vi "Implemeted_Discrete_Controller.vi"(6 "Loop Itr":i32, 8 "Other variables":T1, 9 "systems":T6 {"SysD"."Transport Delay" format="%.2f"; "SysD"."D" format="%#.2g"; "SysD"."C" format="%#.2g"; "SysD"."B" format="%#.2g"; "SysD"."A" format="%#.2g"; "SysD"."properties"."Sampling Time" format="%#.6p"; "SysD"."properties"."Output Delays" format="%.4f"; "SysD"."properties"."Input Delays" format="%.4f"; "sysDo"."Transport Delay" format="%.2f"; "sysDo"."D" format="%#.2g"; "sysDo"."C" format="%#.2g"; "sysDo"."B" format="%#.2g"; "sysDo"."A" format="%#.2g"; "sysDo"."properties"."Sampling Time" format="%#.6p"; "sysDo"."properties"."Output Delays" format="%.4f"; "sysDo"."properties"."Input Delays" format="%.4f"; "sysDi"."Transport Delay" format="%.2f"; "sysDi"."D" format="%#.2g"; "sysDi"."C" format="%#.2g"; "sysDi"."B" format="%#.2g"; "sysDi"."A" format="%#.2g"; "sysDi"."properties"."Sampling Time" format="%#.6p"; "sysDi"."properties"."Output Delays" format="%.4f"; "sysDi"."properties"."Input Delays" format="%.4f"; "sysDC"."transfer function(s)"."delay" format="%.4f"; "sysDC"."transfer function(s)"."Denominator" format="%#_3g"; "sysDC"."transfer function(s)"."Numerator" format="%#_3g"; "sysDC"."properties"."Sampling Time" format="%#.6p"; "sysDC"."properties"."Output Delays" format="%.4f"; "sysDC"."properties"."Input Delays" format="%.4f"}, 10 "Lean Angle":dbl, 11 "Steer Angle":dbl format="%#_13g") -> (2 "Direction":dbl, 3 "Duty Cycle":dbl, 4 "Loop Out":i32)   [LabVIEW 2016]
uses:
  <vilib>/addons/Control Design/_Model Construction/Model Typedefs.llb/CD State Space Model (MIMO).ctl
  <vilib>/addons/Control Design/_Model Construction/Model Typedefs.llb/CD General Elements.ctl
  <vilib>/addons/Control Design/_Model Construction/Model Typedefs.llb/CD Transfer Function Model (MIMO).ctl
  <vilib>/addons/Control Design/_Model Construction/Model Typedefs.llb/CD Transfer Function Model (SISO).ctl
  <vilib>/Analysis/Matrix/Datatypes/RealMatrix.ctl
  <vilib>/Simulation/DiscreteLinear/Implementation/NILVSim Discrete Transfer Function Direct.llb/SIM Discrete Transfer Function Diagram (SISO).vi
  <vilib>/Analysis/baseanly.llb/Real A x B.vi
  <vilib>/Simulation/ContinuousLinear/Implementation/Shared/SIM Transfer Function Support.llb/SIM TransferFunction Normalize to Buffer.vi
  <vilib>/Simulation/DiscreteLinear/Implementation/Shared/SIM Init Discrete States.vi
  <vilib>/Simulation/DiscreteLinear/Implementation/NILVSim Discrete Transfer Function Direct.llb/SIM Transfer Function Direct core (SISO).vi
  <vilib>/Simulation/ContinuousLinear/Implementation/Shared/SIM Transfer Function Support.llb/SIM TransferFunction Normalize.vi
  <vilib>/Simulation/Implementation/Shared/SIM Polynomials.llb/SIM Remove Zero Coefficients (DBL).vi
  <vilib>/Simulation/Implementation/Shared/SIM Polynomials.llb/SIM Divide Polynomials (DBL).vi
  <vilib>/Simulation/Implementation/Shared/SIM BuildSimErr.vi
  <vilib>/Analysis/Matrix/Numeric/Conversions/Matrix To Array - RM.vi
  <vilib>/imath/engines/lvmath2/RunTimeEngine/NodeEndStatement/NIMS_NodeEndStatement_Output.vi
  <instcachedir>/0/NIMS_NodeEndStatement_Output_53EC0D466D134D7ABD903AC30B43404B.lvgen/NIMS_NodeEndStatement_Output_53EC0D466D134D7ABD903AC30B43404B_002.vi
  <vilib>/imath/engines/lvmath2/RunTimeEngine/ErrorHandling/NIMS_Finalize Error.vi
  <vilib>/Analysis/Matrix/Numeric/Subtract/Subtract (Elementwise) - R,RM.vi
  <vilib>/Analysis/Matrix/Numeric/Add/Add - RM,RM.vi
  <vilib>/Simulation/Implementation/XNodeFramework/SimXNode/SimX.xnode
  <vilib>/Analysis/NI_AALBase.lvlib
  <vilib>/Analysis/Matrix/NI_Matrix.lvlib
  <vilib>/addons/Control Design/_Model Construction/NI_LinSys_Model Typedefs.lvlib
panel:
  # "Inputs"
  # "Outputs"
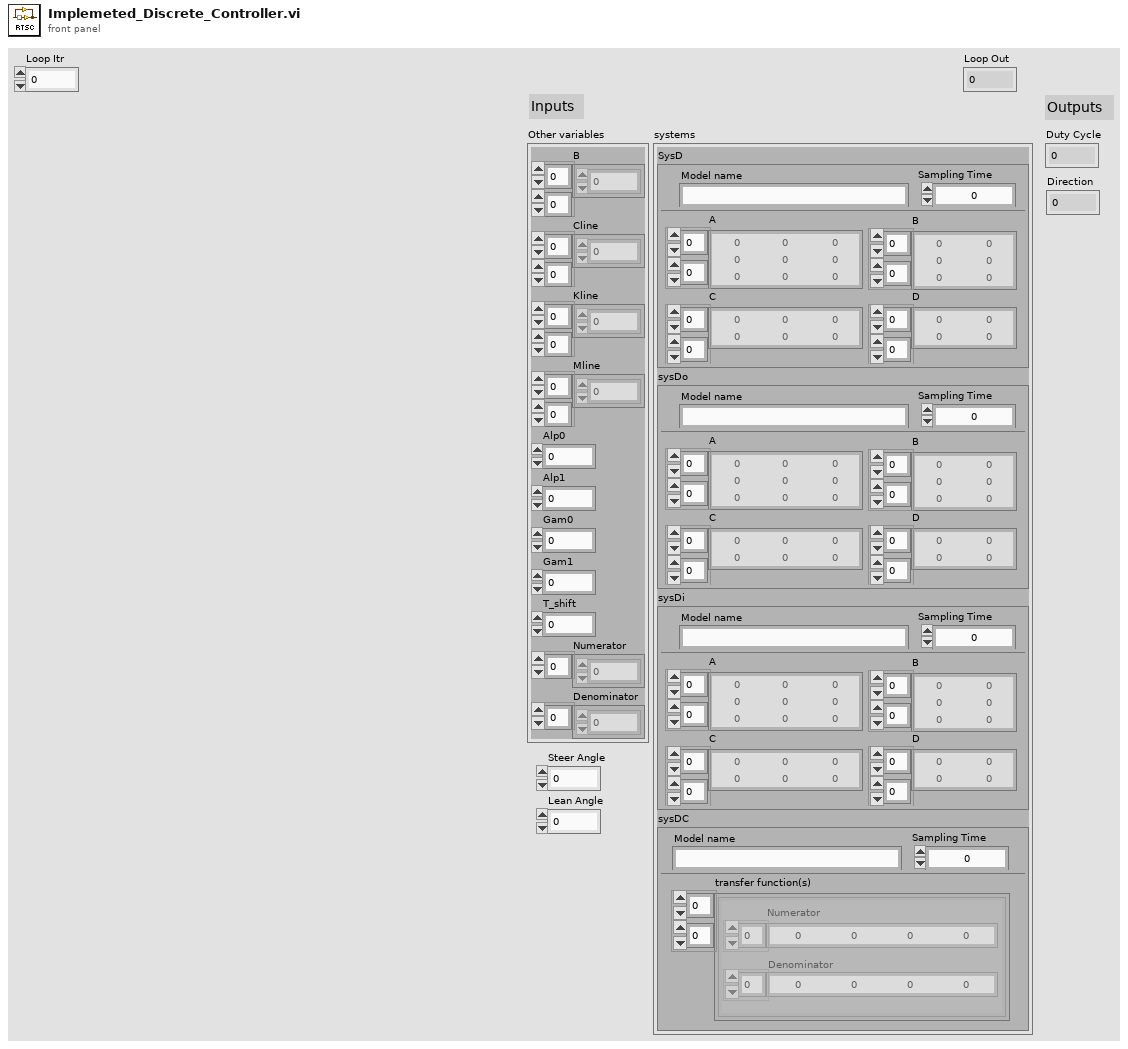
[diagram p1: front panel]
types:
  T1 = cluster{"B":dbl[][], "Cline":dbl[][], "Kline":dbl[][], "Mline":dbl[][], "Alp0":dbl, "Alp1":dbl, "Gam0":dbl, "Gam1":dbl, "T_shift":dbl, "Numerator":dbl[], "Denominator":dbl[]}
  T2 = typedef "NI_LinSys_Model Typedefs.lvlib/CD State Space Model (MIMO).ctl" = cluster{"properties":T3, "A":dbl[][], "B":dbl[][], "C":dbl[][], "D":dbl[][], "StateNames":string[], "Transport Delay":dbl[][]}
  T3 = typedef "NI_LinSys_Model Typedefs.lvlib/CD General Elements.ctl" = cluster{"Model name":string, "Input names":string[], "Output names":string[], "Input Delays":dbl[], "Output Delays":dbl[], "Sampling Time":dbl, "Notes":string}
  T4 = typedef "NI_LinSys_Model Typedefs.lvlib/CD Transfer Function Model (MIMO).ctl" = cluster{"properties":T3, "transfer function(s)":T5[][]}
  T5 = typedef "NI_LinSys_Model Typedefs.lvlib/CD Transfer Function Model (SISO).ctl" = cluster{"Numerator":dbl[], "Denominator":dbl[], "delay":dbl}
  T6 = cluster{"SysD":T2, "sysDo":T2, "sysDi":T2, "sysDC":T4}
  T7 = typedef "NI_Matrix.lvlib/RealMatrix.ctl" = dbl[][]
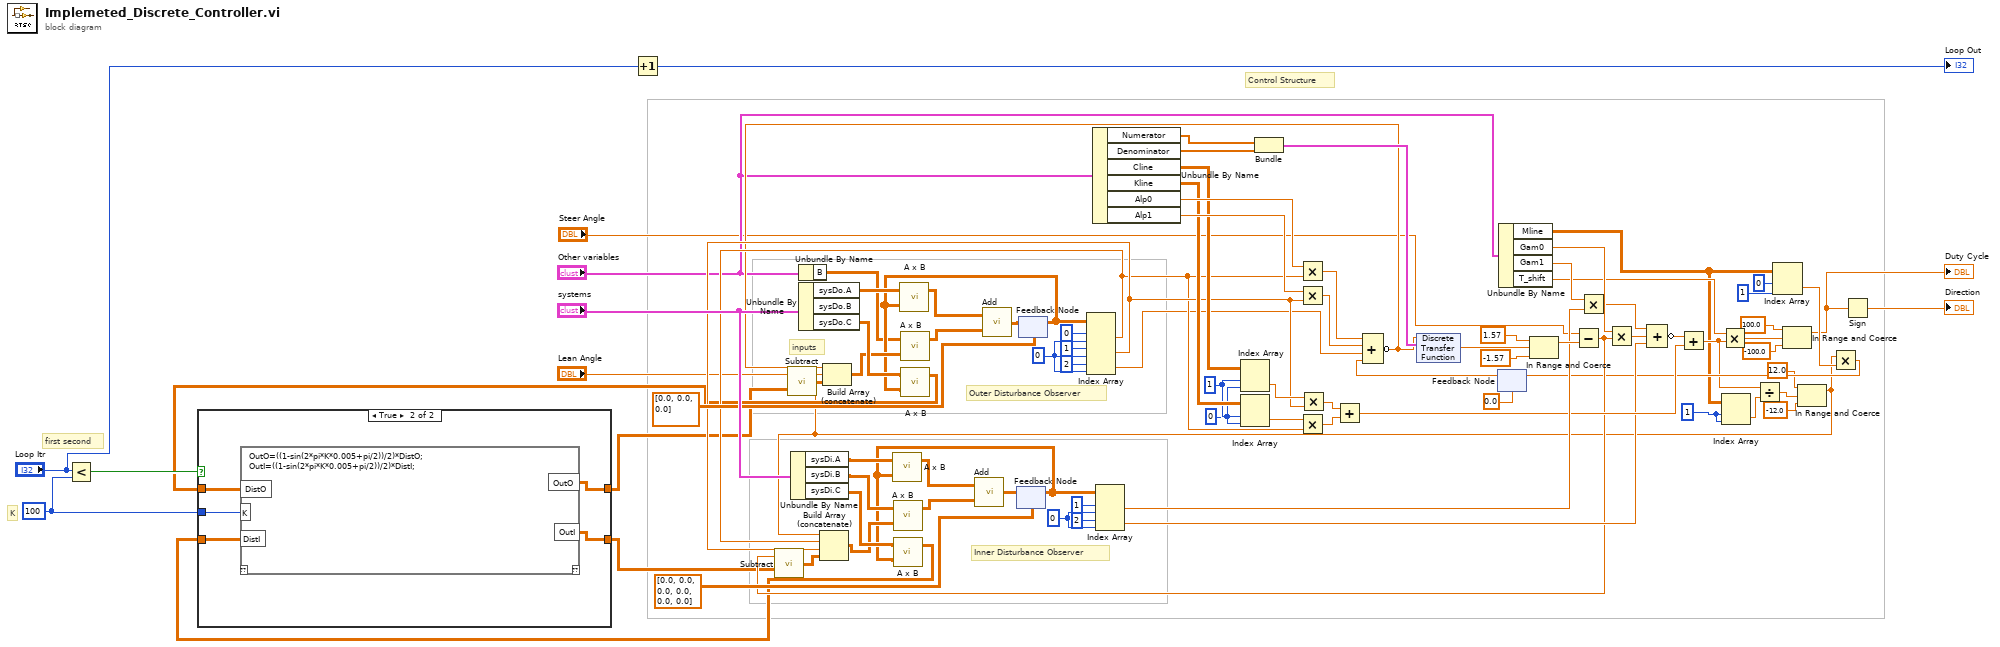
[diagram p0: block diagram]
diagram:
  w5 = 1 ("index (row)")
  w16 = 100
  w57 = 0 ("index (row) 9")
  w58 = 1 ("index (row) 8")
  w67 = 0 ("index (row) 5")
  w72 = 0 ("index (row)")
  # "K"
  # "first second"
  # "Control Structure"
  # "Outer Disturbance Observer"
  # "Inner Disturbance Observer"
  # "inputs"
  n1 = Less?(x="Loop Itr", y=w16) -> (x < y?=w15:bool)
  n2 = Increment(x="Loop Itr") -> (x+1=→"Loop Out":i32)
  n3 = Unbundle By Name ("Unbundle By Name 2")("systems") -> ("sysDi.A"=w80:dbl[][], "sysDi.B"=w79:dbl[][], "sysDi.C"=w78:dbl[][])
  n4 = Unbundle By Name("Other variables") -> ("B"=w26:dbl[][])
  n5 = Unbundle By Name("systems") -> ("sysDo.A"=w88:dbl[][], "sysDo.C"=w84:dbl[][])  [unwired: 1 out]
  n6 = feedback #1 ("Feedback Node 2")(T7 [[0.0], [0.0], [0.0], [0.0], [0.0], [0.0]] ("A + B")) -> (w68:T7)
  n7 = call-poly <vilib>:"A x B.vi"("B"=w68, "A"=w80) -> ("A x B"=w82:T7)  [unwired: 1 out]
  n8 = call-poly <vilib>:"A x B.vi"("B"=w68, "A"=w78) -> ("A x B"=w10:T7)  [unwired: 1 out]
  n9 = feedback #2(T7 [[0.0], [0.0], [0.0]] ("A + B")) -> (w73:T7)
  n10 = call-poly <vilib>:"A x B.vi"("B"=w73, "A"=w88) -> ("A x B"=w86:T7)  [unwired: 1 out]
  n11 = call-poly <vilib>:"A x B.vi"("B"=w73, "A"=w84) -> ("A x B"=w12:T7)  [unwired: 1 out]
  n12 = case shown="True" w15 {
    tunnel: w16 -> [_ w98]
    tunnel: w12 -> [w93 w97]
    tunnel: [w93 w96] -> w11
    tunnel: w10 -> [w92 w95]
    tunnel: [w92 w94] -> w9
    frame False {
    }
    frame True {
      n13 = mathscript code="OutO=((1-sin(2*pi*K*0.005+pi/2))/2)*DistO;\nOutI=((1-sin(2*pi*K*0.005+pi/2))/2)*DistI;"("DistO"=w97, "DistI"=w95, "K"=w98) -> ("OutI"=w94:dbl[][], "OutO"=w96:dbl[][])  [unwired: 1 in, 1 out]
    }
  }
  n14 = call-poly <vilib>:"Subtract.vi"("Real Matrix A"=w11, "Real Scalar c"="Lean Angle") -> ("c - A"=w75:T7)
  n15 = Index Array ("Get Matrix Elements")(array=w73, index (row) #1=0 ("index (row) 2"), index (col) #1=w72, index (row) #2=1 ("index (row) 3"), index (col) #2=w72, index (row) #3=2 ("index (row) 4"), index (col) #3=w72) -> (element #1=w53:dbl, element #2=w54:dbl, element #3=w50:dbl)
  n16 = Unbundle By Name ("Unbundle By Name 3")("Other variables") -> ("Numerator"=w30:dbl[], "Denominator"=w29:dbl[], "Cline"=w60:dbl[][], "Kline"=w59:dbl[][], "Alp0"=w63:dbl, "Alp1"=w64:dbl)
  n17 = Index Array ("Get Matrix Elements 2")(array=w68, index (row) #1=1 ("index (row) 6"), index (col) #1=w67, index (row) #2=2 ("index (row) 7"), index (col) #2=w67) -> (element #1=w42:dbl, element #2=w35:dbl)
  n18 = Index Array ("Get Matrix Elements 3")(array=w60, index (row)=w58, index (col)=w57) -> (element=w55:dbl)
  n19 = Index Array ("Get Matrix Elements 4")(array=w59, index (row)=w58, index (col)=w57) -> (element=w56:dbl)
  n20 = Bundle("Numerator"=w30, "Denominator"=w29) -> (w28:cluster{"Numerator":dbl[], "Denominator":dbl[]})  [unwired: 1 in]
  n21 = Multiply ("Multiply 4")(x=w63, y=w53) -> (x*y=w62:dbl)
  n22 = Multiply ("Multiply 5")(x=w64, y=w54) -> (x*y=w61:dbl)
  n23 = Multiply ("Multiply 7")(x=w56, y=w53) -> (x*y=w51:dbl)
  n24 = Multiply ("Multiply 6")(x=w55, y=w54) -> (x*y=w52:dbl)
  n25 = Add ("Add.vi 3")(x=w52, y=w51) -> (x+y=w40:dbl)
  n26 = feedback #3(0.0 ("output y(k)")) -> (w23:dbl)
  n27 = Compound Arithmetic op=ADD(w62, w61, w50, w23) -> (invert w27:dbl)
  n28 = xnode ("Discrete Transfer Function")("input u(k)"=w27, "Transfer Function"=w28) -> ("output y(k)"=w22:dbl)  [unwired: 2 in, 1 out]
  n29 = Unbundle By Name ("Unbundle By Name 5")("Other variables") -> ("Mline"=w6:dbl[][], "Gam0"=w46:dbl, "Gam1"=w43:dbl, "T_shift"=w39:dbl)
  n30 = In Range and Coerce(upper limit=1.57, x=w22, lower limit=-1.57 ("upper limit 2")) -> (coerced(x)=w47:dbl)  [unwired: 1 out]
  n31 = Subtract(x="Steer Angle", y=w47) -> (x-y=w31:dbl)
  n32 = call-poly <vilib>:"Subtract.vi"("Real Matrix A"=w9, "Real Scalar c"=w31) -> ("c - A"=w76:T7)
  n33 = Multiply ("Multiply 9")(x=w43, y=w42) -> (x*y=w36:dbl)
  n34 = Multiply ("Multiply 8")(x=w46, y=w31) -> (x*y=w37:dbl)
  n35 = Compound Arithmetic op=ADD ("Compound Arithmetic 2")(w36, w37, w35) -> (invert w41:dbl)
  n36 = Add ("Add.vi 4")(x=w41, y=w40) -> (x+y=w8:dbl)
  n37 = Multiply ("Multiply 10")(x=w39, y=w8) -> (x*y=w38:dbl)
  n38 = Index Array ("Get Matrix Elements 5")(array=w6, index (row)=w5, index (col)=w5) -> (element=w7:dbl)
  n39 = Divide(x=w8, y=w7) -> (x/y=w3:dbl)
  n40 = Index Array ("Get Matrix Elements 5")(array=w6, index (row)=0, index (col)=1 ("index (row) 10")) -> (element=w32:dbl)
  n41 = In Range and Coerce ("In Range and Coerce 2")(upper limit=100.0 ("upper limit 3"), x=w38, lower limit=-100.0 ("upper limit 4")) -> (coerced(x)=w17:dbl)  [unwired: 1 out]
  "Duty Cycle" <- w17
  n42 = In Range and Coerce ("In Range and Coerce 2")(upper limit=12.0 ("lower limit"), x=w3, lower limit=-12.0) -> (coerced(x)=w4:dbl)  [unwired: 1 out]
  n43 = Build Array (concatenate) ("Build Matrix")(w4, w53, w54, w76) -> (w77:T7)
  n44 = Build Array (concatenate) ("Build Matrix 2")(w27, w4, w75) -> (w74:T7)
  n45 = call-poly <vilib>:"A x B.vi"("B"=w77, "A"=w79) -> ("A x B"=w83:T7)  [unwired: 1 out]
  n46 = call-poly <vilib>:"A x B.vi"("B"=w74, "A"=w26) -> ("A x B"=w87:T7)  [unwired: 1 out]
  n47 = call-poly <vilib>:"Add.vi"("Real Matrix B"=w83, "Real Matrix A"=w82) -> ("A + B"=w81:T7)
  n48 = call-poly <vilib>:"Add.vi"("Real Matrix B"=w87, "Real Matrix A"=w86) -> ("A + B"=w85:T7)
  n49 = feedback-in #1 ("3")(w81) -> ()
  n50 = feedback-in #2 ("2")(w85) -> ()
  n51 = Multiply ("Multiply 11")(x=w4, y=w32) -> (x*y=w24:dbl)
  n52 = feedback-in #3(w24) -> ()
  n53 = Sign(1:w17) -> (0:→"Direction":dbl)
